vi "Cryostat Temperature Control.vi"() -> ()   [LabVIEW 2012]
panel:
  out "X Scale.Range:Minimum":dbl
  out "X Scale.Range:Maximum":dbl
  out "double precision float":dbl
  in  "Milliseconds between update":u32=200
  in  "Clear":bool
  out "Temperature":cluster{"Temperature":dbl, "Temperature":dbl}(graph)
  in  "Control Type Set":u8(ring) items=["Off", "PID", "Man", "Table", "RampP"]
  out "Loop 2 Control Type":string
  in  "Set Control Method":u8(ring) items=["Off", "PID", "Man", "Table", "RampP"]
  in  "Loop Set Control Type":bool
  out "Set Temperature":dbl format="%.3f"
  in  "Set Temp":bool
  out "Loop 1 Control Method":string
  in  "Loop 1 Type?":bool
  in  "Control Off":bool
  in  "Control On":bool
  out "Status of \nControl Loops":string
  in  "Desired Temp":dbl format="%#.3g"
  out "Temperature B":dbl format="%.3f"
  out "Temperature A":dbl format="%.3f"
  out "Sensor Name":string
  in  "Set Temperature Units":u8(ring) items=["K", "C", "F", "Sensor"]
  in  "Set Sensor Index":u8=3 step=1
  out "Sensor Index #":u8=3 step=1
  out "Units":string
  out "Input Name":string
  in  "Channel":bool
  in  "error in (no error)":errorcluster
  out "error out":T1
  in  "Read":bool
  in  "Set":bool
  in  "Exit":bool
  in  "stop":bool
  # "Temperature Settings"
  # "Sensor Settings"
  # "I believe the default settings\nfor the controller are:\nCh A - Sensor 14 (AKA \"None\")\nCh B - Sensor 13 (AKA \"None\")\n-Mitch 7-30-09"
  # "Current Settings"
  # "Control Loops On/Off"
  # "Loop 1"
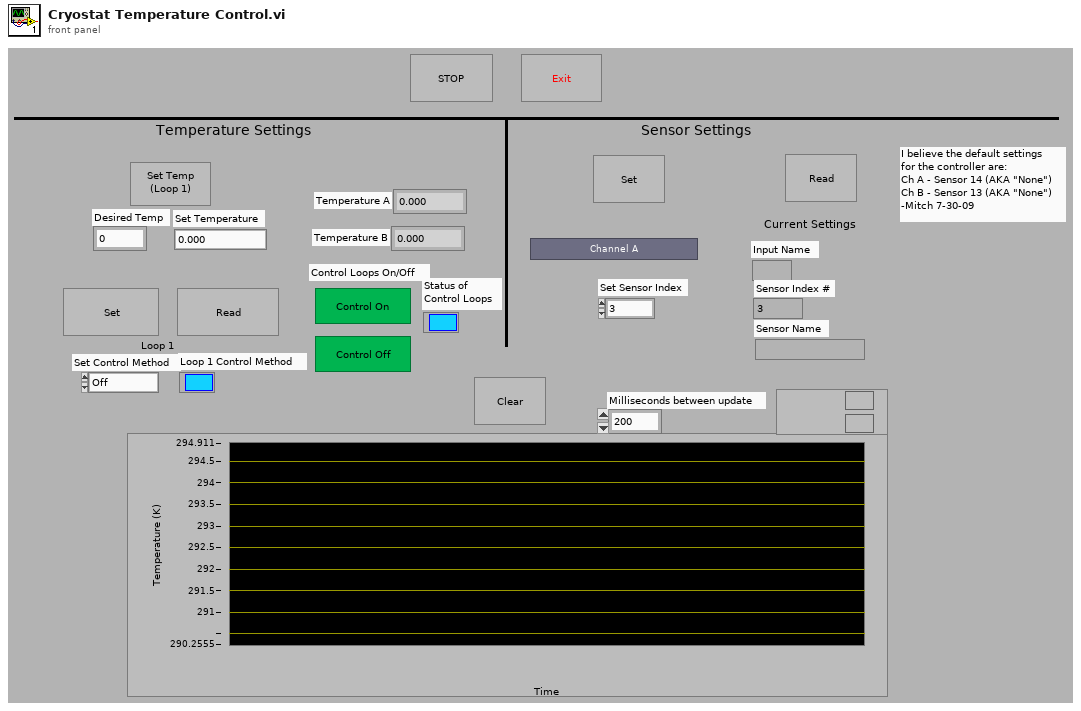
[diagram p1: front panel]
types:
  T1 = cluster{"status":bool, "code 2":i32, "source 2":string}
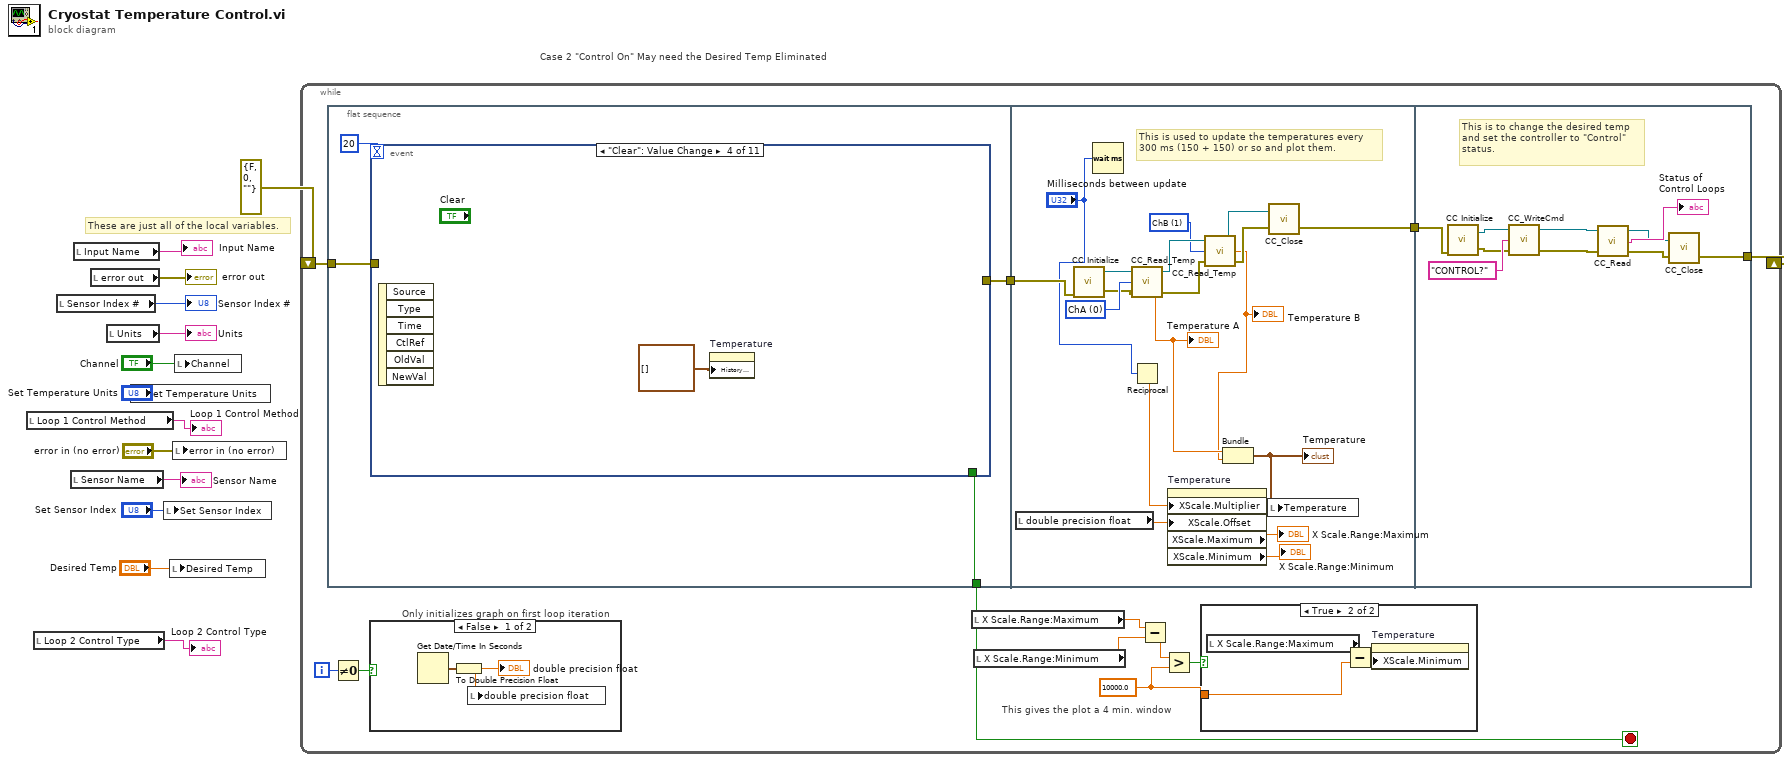
[diagram p0: block diagram]
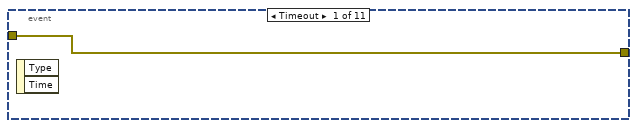
[diagram p4: hidden frame]
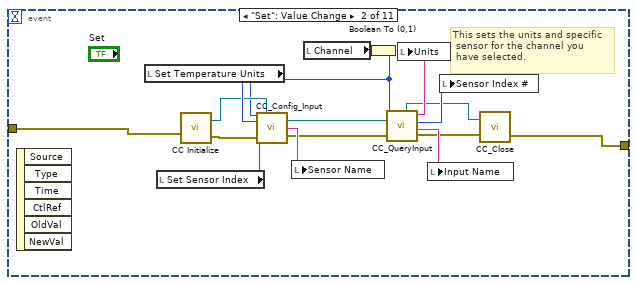
[diagram p5: hidden frame]
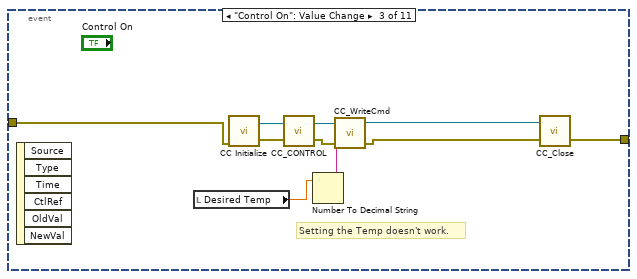
[diagram p6: hidden frame]
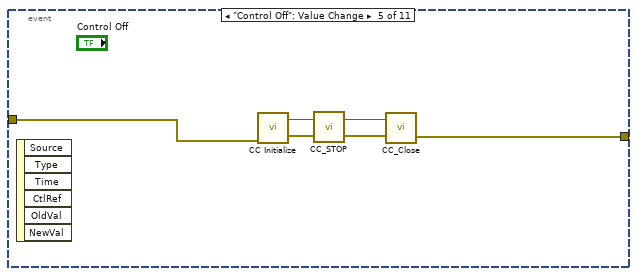
[diagram p7: hidden frame]
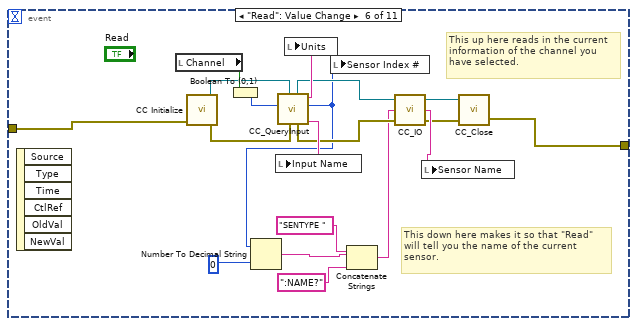
[diagram p8: hidden frame]
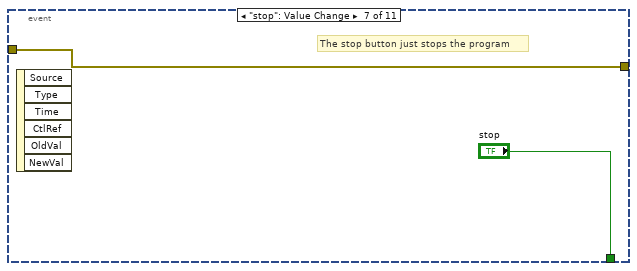
[diagram p9: hidden frame]
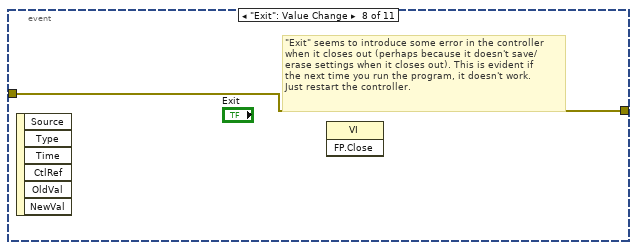
[diagram p10: hidden frame]
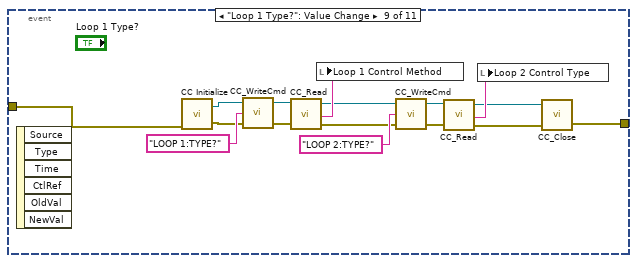
[diagram p11: hidden frame]
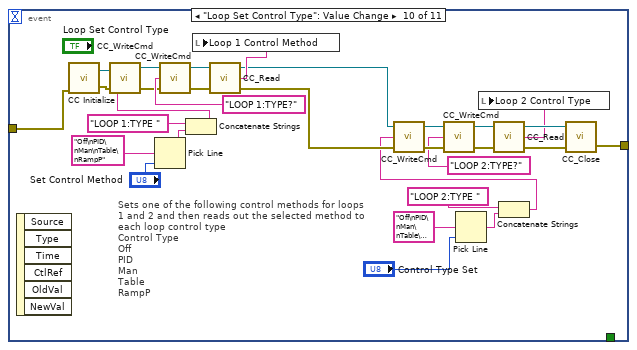
[diagram p12: hidden frame]
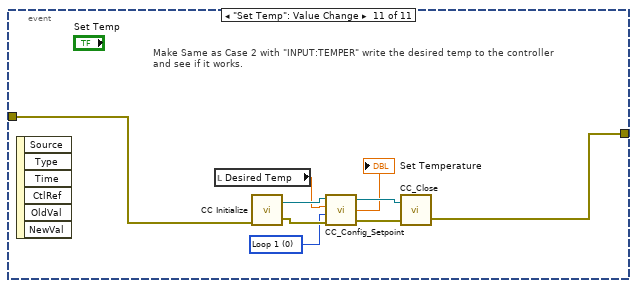
[diagram p13: hidden frame]
diagram:
  # "Case 2 \"Control On\" May need the Desired Temp Eliminated"
  # "These are just all of the local variables."
  n1 = local read "Loop 1 Control Method"() -> (→"Loop 1 Control Method":string)
  n2 = local read "Loop 2 Control Type"() -> (→"Loop 2 Control Type":string)
  n3 = local read "Sensor Index #"() -> (→"Sensor Index #":u8)
  n4 = local read "Sensor Name"() -> (→"Sensor Name":string)
  n5 = local read "Input Name"() -> (→"Input Name":string)
  n6 = local read "error out"() -> (→"error out":T1)
  n7 = local read "Units"() -> (→"Units":string)
  n8 = local write "Set Temperature Units"("Set Temperature Units") -> ()
  n9 = local write "Set Sensor Index"("Set Sensor Index") -> ()
  n10 = local write "Desired Temp"("Desired Temp") -> ()
  n11 = local write "error in (no error)"("error in (no error)") -> ()
  n12 = local write "Channel"("Channel") -> ()
  n13 = while {
    shift-right: [w22] -> _
    shift-left: errorcluster {"status"=FALSE, "code"=0, "source"=""} ("error out") -> [w23]
    i -> [w20]
    stop <- w25 stop-if-true
    w14 = 10000.0 ("y")
    # "Only initializes graph on first loop iteration"
    # "This gives the plot a 4 min. window"
    n14 = flat-sequence {
      tunnel: [w31] -> w25
      tunnel: [w33] -> w24
      tunnel: w23 -> [w32]
      tunnel: w24 -> [w155]
      tunnel: [w154] -> w21
      tunnel: [w173] -> w22
      tunnel: w21 -> [w172]
      frame #0 {
        n15 = event shown="[3] \"Clear\": Value Change" {
          selector: _ -> [_ _ _ _ _ _ _ _ _ _ _]
          dyn-events: _ -> [_ _ _ _ _ _ _ _ _ _ _]
          timeout: 20 -> [_ _ _ _ _ _ _ _ _ _ _]
          tunnel: [_ _ _ _ _ _ "stop" _ _ _ _] -> w31
          tunnel: [w35 w37 w59 _ w64 w70 w88 w90 w100 w134 w144] -> w33
          tunnel: w32 -> [w35 w36 w58 _ w63 w69 w88 w90 w101 w133 w145]
          event Timeout {
            n16 = event-data() -> ()  [unwired: 3 out]
          }
          event "Set": Value Change {
            # "This sets the units and specific\n sensor for the channel you\n have selected."
            n17 = event-data() -> ()  [unwired: 7 out]
            n18 = local read "Set Temperature Units"() -> (w49:u8)
            n19 = local read "Set Sensor Index"() -> (w51:u8)
            n20 = call "CC Initialize.vi"("error in (no error)"=w36) -> ("error out"=w40:errorcluster, "VISA out"=w39:refnum<visa-resource-name>)  [unwired: 2 in, 1 out]
            n21 = local read "Channel"() -> (w48:bool)
            n22 = Boolean To (0,1)(Boolean=w48) -> (0, 1=w38:i16)
            n23 = call "CC_Config_Input.vi"("Input"=w38, "VISA In"=w39, "Units"=w49, "Sensor Index"=w51, "error in (no error)"=w40) -> ("VISA Out"=w41:refnum<visa-resource-name>, "error out"=w42:errorcluster, "Sensor Name"=w50:string)  [unwired: 1 in, 7 out]
            n24 = local write "Sensor Name"(w50) -> ()
            n25 = call "CC_QueryInput.vi"("error in (no error)"=w42, "VISA In"=w41, "Input"=w38) -> ("Name"=w45:string, "Sensor Index"=w46:u8, "Units"=w47:string, "error out"=w44:errorcluster, "VISA Out"=w43:refnum<visa-resource-name>)  [unwired: 4 out]
            n26 = local write "Units"(w47) -> ()
            n27 = local write "Input Name"(w45) -> ()
            n28 = local write "Sensor Index #"(w46) -> ()
            n29 = call "CC_Close.vi"("error in (no error)"=w44, "VISA In"=w43) -> ("error out"=w37:errorcluster)  [unwired: 1 out]
          }
          event "Control On": Value Change {
            # "Setting the Temp doesn't work."
            n30 = event-data() -> ()  [unwired: 7 out]
            n31 = local read "Desired Temp"() -> (w54:dbl)
            n32 = call "CC Initialize.vi"("error in (no error)"=w58) -> ("error out"=w61:errorcluster, "VISA out"=w60:refnum<visa-resource-name>)  [unwired: 3 in]
            n33 = call "CC_CONTROL.vi"("error in (no error)"=w61, "VISA In"=w60) -> ("error out"=w57:errorcluster, "VISA Out"=w56:refnum<visa-resource-name>)
            n34 = Number To Decimal String(number=w54) -> (decimal integer string=w55:string)  [unwired: 1 out]
            n35 = call "CC_WriteCmd.vi"("error in (no error)"=w57, "Output Command"=w55, "VISA In"=w56) -> ("error out"=w52:errorcluster, "VISA Out"=w53:refnum<visa-resource-name>)  [unwired: 1 out]
            n36 = call "CC_Close.vi"("error in (no error)"=w52, "VISA In"=w53) -> ("error out"=w59:errorcluster)  [unwired: 1 out]
          }
          event "Clear": Value Change {
            n37 = event-data() -> ()  [unwired: 7 out]
            n38 = property on="Temperature" class="WFChart (strict)"("History Data"=cluster{"Temperature":dbl, "Temperature":dbl}[] []) -> ()  [unwired: 2 in, 2 out]
          }
          event "Control Off": Value Change {
            n39 = event-data() -> ()  [unwired: 7 out]
            n40 = call "CC Initialize.vi"("error in (no error)"=w63) -> ("error out"=w67:errorcluster, "VISA out"=w68:refnum<visa-resource-name>)  [unwired: 3 in]
            n41 = call "CC_STOP.vi"("error in (no error)"=w67, "VISA In"=w68) -> ("error out"=w65:errorcluster, "VISA Out"=w66:refnum<visa-resource-name>)
            n42 = call "CC_Close.vi"("error in (no error)"=w65, "VISA In"=w66) -> ("error out"=w64:errorcluster)  [unwired: 1 out]
          }
          event "Read": Value Change {
            # "This up here reads in the current\ninformation of the channel you \nhave selected."
            # "This down here makes it so that \"Read\"\nwill tell you the name of the current\nsensor."
            n43 = event-data() -> ()  [unwired: 7 out]
            n44 = local read "Channel"() -> (w87:bool)
            n45 = call "CC Initialize.vi"("error in (no error)"=w69) -> ("error out"=w83:errorcluster, "VISA out"=w84:refnum<visa-resource-name>)  [unwired: 2 in, 1 out]
            n46 = Boolean To (0,1)(Boolean=w87) -> (0, 1=w72:i16)
            n47 = call "CC_QueryInput.vi"("error in (no error)"=w83, "VISA In"=w84, "Input"=w72) -> ("Name"=w85:string, "Sensor Index"=w71:u8, "Units"=w86:string, "error out"=w78:errorcluster, "VISA Out"=w77:refnum<visa-resource-name>)  [unwired: 4 out]
            n48 = Number To Decimal String(number=w71, width (-)=0) -> (decimal integer string=w79:string)
            n49 = local write "Input Name"(w85) -> ()
            n50 = local write "Units"(w86) -> ()
            n51 = local write "Sensor Index #"(w71) -> ()
            n52 = Concatenate Strings("SENTYPE ", w79, ":NAME?") -> (w76:string)
            n53 = call "CC_IO.vi"("error in (no error)"=w78, "Output Command"=w76, "VISA In"=w77) -> ("error out"=w74:errorcluster, "Input String"=w75:string, "VISA out"=w73:refnum<visa-resource-name>)
            n54 = local write "Sensor Name"(w75) -> ()
            n55 = call "CC_Close.vi"("error in (no error)"=w74, "VISA In"=w73) -> ("error out"=w70:errorcluster)  [unwired: 1 out]
          }
          event "stop": Value Change {
            # "The stop button just stops the program"
            n56 = event-data() -> ()  [unwired: 7 out]
          }
          event "Exit": Value Change {
            # "\"Exit\" seems to introduce some error in the controller\nwhen it closes out (perhaps because it doesn't save/\nerase settings when it closes out). This is evident if \nthe next time you run the program, it doesn't work.\nJust restart the controller."
            n57 = event-data() -> ()  [unwired: 7 out]
            n58 = invoke class="VI" method="FP.Close"() -> ()  [unwired: 3 in, 3 out]
          }
          event "Loop 1 Type?": Value Change {
            n59 = event-data() -> ()  [unwired: 7 out]
            n60 = call "CC Initialize.vi"("error in (no error)"=w101) -> ("error out"=w103:errorcluster, "VISA out"=w102:refnum<visa-resource-name>)  [unwired: 3 in]
            n61 = call "CC_WriteCmd.vi"("error in (no error)"=w103, "Output Command"="LOOP 1:TYPE?" ("Output Command   2"), "VISA In"=w102) -> ("error out"=w106:errorcluster, "VISA Out"=w105:refnum<visa-resource-name>)  [unwired: 1 out]
            n62 = call "CC_Read.vi"("error in (no error)"=w106, "VISA In"=w105) -> ("error out"=w94:errorcluster, "Input String"=w99:string, "VISA Out"=w93:refnum<visa-resource-name>)  [unwired: 1 out]
            n63 = local write "Loop 1 Control Method"(w99) -> ()
            n64 = call "CC_WriteCmd.vi"("error in (no error)"=w94, "Output Command"="LOOP 2:TYPE?" ("Output Command   2"), "VISA In"=w93) -> ("error out"=w95:errorcluster, "VISA Out"=w96:refnum<visa-resource-name>)  [unwired: 1 out]
            n65 = call "CC_Read.vi"("error in (no error)"=w95, "VISA In"=w96) -> ("error out"=w91:errorcluster, "Input String"=w98:string, "VISA Out"=w92:refnum<visa-resource-name>)  [unwired: 1 out]
            n66 = local write "Loop 2 Control Type"(w98) -> ()
            n67 = call "CC_Close.vi"("error in (no error)"=w91, "VISA In"=w92) -> ("error out"=w100:errorcluster)  [unwired: 1 out]
          }
          event "Loop Set Control Type": Value Change {
            # "Sets one of the following control methods for loops\n1 and 2 and then reads out the selected method to\neach loop control type\nControl Type\nOff\nPID\nMan\nTable\nRampP"
            n68 = event-data() -> ()  [unwired: 7 out]
            n69 = call "CC Initialize.vi"("error in (no error)"=w133) -> ("error out"=w135:errorcluster, "VISA out"=w136:refnum<visa-resource-name>)  [unwired: 3 in]
            n70 = Pick Line(multi-line string="Off\nPID\nMan\nTable\nRampP", line index="Set Control Method") -> (output string=w129:string)  [unwired: 1 out]
            n71 = Concatenate Strings("LOOP 1:TYPE " ("Output Command   2"), w129) -> (w130:string)
            n72 = call "CC_WriteCmd.vi"("error in (no error)"=w135, "Output Command"=w130, "VISA In"=w136) -> ("error out"=w125:errorcluster, "VISA Out"=w124:refnum<visa-resource-name>)  [unwired: 1 out]
            n73 = call "CC_WriteCmd.vi"("error in (no error)"=w125, "Output Command"="LOOP 1:TYPE?" ("Output Command   2"), "VISA In"=w124) -> ("error out"=w123:errorcluster, "VISA Out"=w122:refnum<visa-resource-name>)  [unwired: 1 out]
            n74 = call "CC_Read.vi"("error in (no error)"=w123, "VISA In"=w122) -> ("error out"=w114:errorcluster, "Input String"=w132:string, "VISA Out"=w115:refnum<visa-resource-name>)  [unwired: 1 out]
            n75 = local write "Loop 1 Control Method"(w132) -> ()
            n76 = Pick Line(multi-line string="Off\nPID\nMan\nTable\nRampP", line index="Control Type Set") -> (output string=w111:string)  [unwired: 1 out]
            n77 = Concatenate Strings("LOOP 2:TYPE " ("Output Command   2"), w111) -> (w108:string)
            n78 = call "CC_WriteCmd.vi"("error in (no error)"=w114, "Output Command"=w108, "VISA In"=w115) -> ("error out"=w121:errorcluster, "VISA Out"=w120:refnum<visa-resource-name>)  [unwired: 1 out]
            n79 = call "CC_WriteCmd.vi"("error in (no error)"=w121, "Output Command"="LOOP 2:TYPE?" ("Output Command   2"), "VISA In"=w120) -> ("error out"=w119:errorcluster, "VISA Out"=w118:refnum<visa-resource-name>)  [unwired: 1 out]
            n80 = call "CC_Read.vi"("error in (no error)"=w119, "VISA In"=w118) -> ("error out"=w117:errorcluster, "Input String"=w113:string, "VISA Out"=w116:refnum<visa-resource-name>)  [unwired: 1 out]
            n81 = local write "Loop 2 Control Type"(w113) -> ()
            n82 = call "CC_Close.vi"("error in (no error)"=w117, "VISA In"=w116) -> ("error out"=w134:errorcluster)  [unwired: 1 out]
          }
          event "Set Temp": Value Change {
            w137 = u8 0 items=["Loop 1", "Loop 2"] ("Output")
            # "Make Same as Case 2 with \"INPUT:TEMPER\" write the desired temp to the controller\nand see if it works."
            n83 = event-data() -> ()  [unwired: 7 out]
            n84 = local read "Desired Temp"() -> (w138:dbl)
            n85 = call "CC Initialize.vi"("error in (no error)"=w145) -> ("error out"=w143:errorcluster, "VISA out"=w140:refnum<visa-resource-name>)  [unwired: 3 in]
            n86 = call "CC_Config_Setpoint.vi"("error in (no error)"=w143, "Output"=w137, "Set Point"=w138, "VISA In"=w140) -> ("error out"=w142:errorcluster, "Set Point Returned"=→"Set Temperature":sgl, "VISA Out"=w141:refnum<visa-resource-name>)
            n87 = call "CC_Close.vi"("error in (no error)"=w142, "VISA In"=w141) -> ("error out"=w144:errorcluster)  [unwired: 1 out]
          }
        }
      }
      frame #1 {
        w156 = u8 1 items=["ChA", "ChB", "ChC", "ChD"] ("Input")
        w163 = u8 0 items=["ChA", "ChB", "ChC", "ChD"] ("Set Input")
        # "This is used to update the temperatures every \n300 ms (150 + 150) or so and plot them."
        n88 = local read "double precision float"() -> (w148:dbl)
        n89 = call "CC Initialize.vi"("error in (no error)"=w155) -> ("error out"=w162:errorcluster, "VISA out"=w161:refnum<visa-resource-name>)  [unwired: 3 in]
        n90 = Wait (ms)(milliseconds to wait="Milliseconds between update") -> ()  [unwired: 1 out]
        n91 = call "CC_Read_Temp.vi"("error in (no error)"=w162, "Input"=w163, "VISA In"=w161) -> ("error out"=w159:errorcluster, "Temperature"=w153:dbl, "VISA Out"=w160:refnum<visa-resource-name>)
        "Temperature A" <- w153
        n92 = Reciprocal(x="Milliseconds between update") -> (1/x=w149:dbl)
        n93 = property on="Temperature" class="WFChart (strict)"("XScale.Multiplier"=w149, "XScale.Offset"=w148) -> ("XScale.Maximum"=→"X Scale.Range:Maximum":dbl, "XScale.Minimum"=→"X Scale.Range:Minimum":dbl)  [unwired: 2 in, 2 out]
        n94 = call "CC_Read_Temp.vi"("error in (no error)"=w159, "Input"=w156, "VISA In"=w160) -> ("error out"=w158:errorcluster, "Temperature"=w152:dbl, "VISA Out"=w157:refnum<visa-resource-name>)
        "Temperature B" <- w152
        n95 = Bundle("Temperature"=w153, "Temperature"=w152) -> (w151:cluster{"Temperature":dbl, "Temperature":dbl})  [unwired: 1 out]
        "Temperature" <- w151
        n96 = local write "Temperature"(w151) -> ()
        n97 = call "CC_Close.vi"("error in (no error)"=w158, "VISA In"=w157) -> ("error out"=w154:errorcluster)  [unwired: 1 out]
      }
      frame #2 {
        # "This is to change the desired temp\nand set the controller to \"Control\"\nstatus."
        n98 = call "CC Initialize.vi"("error in (no error)"=w172) -> ("error out"=w165:errorcluster, "VISA out"=w164:refnum<visa-resource-name>)  [unwired: 3 in]
        n99 = call "CC_WriteCmd.vi"("error in (no error)"=w165, "Output Command"="CONTROL?" ("Output Command   2"), "VISA In"=w164) -> ("error out"=w170:errorcluster, "VISA Out"=w169:refnum<visa-resource-name>)  [unwired: 1 out]
        n100 = call "CC_Read.vi"("error in (no error)"=w170, "VISA In"=w169) -> ("error out"=w167:errorcluster, "Input String"=→"Status of \nControl Loops":string, "VISA Out"=w166:refnum<visa-resource-name>)  [unwired: 1 out]
        n101 = call "CC_Close.vi"("error in (no error)"=w167, "VISA In"=w166) -> ("error out"=w173:errorcluster)  [unwired: 1 out]
      }
    }
    n102 = Not Equal To 0?(x=w20) -> (x != 0?=w19:bool)
    n103 = case shown="False" w19 {
      frame False {
        n104 = Get Date/Time In Seconds() -> (seconds since 1Jan1904=w30:timestamp)
        n105 = To Double Precision Float(number=w30) -> (double precision float=w29:dbl)
        "double precision float" <- w29
        n106 = local write "double precision float"(w29) -> ()
      }
      frame True {
        # "Do nothing"
      }
    }
    n107 = local read "X Scale.Range:Maximum"() -> (w18:dbl)
    n108 = local read "X Scale.Range:Minimum"() -> (w17:dbl)
    n109 = Subtract(x=w18, y=w17) -> (x-y=w15:dbl)
    n110 = Greater?(x=w15, y=w14) -> (0:w16:bool)
    n111 = case shown="True" w16 {
      tunnel: w14 -> [_ w26]
      frame False {
      }
      frame True {
        n112 = local read "X Scale.Range:Maximum"() -> (w27:dbl)
        n113 = Subtract(x=w27, y=w26) -> (x-y=w28:dbl)
        n114 = property on="Temperature" class="WFChart (strict)"("XScale.Minimum"=w28) -> ()  [unwired: 2 in, 2 out]
      }
    }
  }
